vi "ComputeColorROI.vi"(1 "Array":dbl[](array[numeric])) -> (0 "Rectangle":T1 {"Rotation" min=-90.0 max=90.0 step=1.0 format="%.2f"; "Left" scale=0.0..1024.0; "Right" scale=0.0..1024.0})   [LabVIEW 2017]
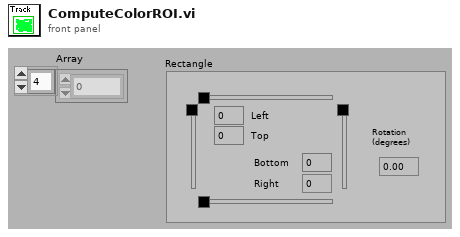
[diagram p1: front panel]
types:
  T1 = typedef "IMAQ Rectangle" = cluster{"Left":i32, "Top":i32, "Right":i32, "Bottom":i32, "Rotation":dbl}
  T2 = cluster{"Numeric":dbl, "Numeric":dbl, "Numeric":dbl, "Numeric":dbl}
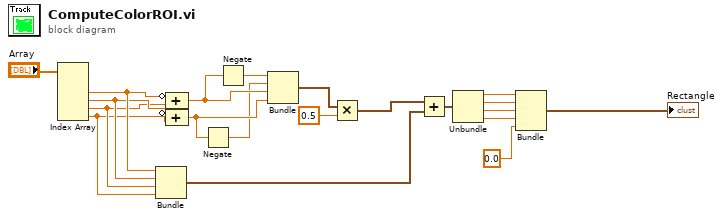
[diagram p0: block diagram]
diagram:
  n1 = Index Array(array="Array") -> (element #2=w10:dbl, element #3=w9:dbl, element #4=w8:dbl, element #5=w7:dbl)  [unwired: 5 in, 1 out]
  n2 = Bundle("Numeric"=w10, "Numeric"=w9, "Numeric"=w8, "Numeric"=w7) -> (w5:T2)  [unwired: 1 in]
  n3 = Compound Arithmetic op=ADD(invert w10, w8) -> (w15:dbl)
  n4 = Compound Arithmetic op=ADD(invert w9, w7) -> (w13:dbl)
  n5 = Negate(x=w13) -> (-x=w12:dbl)
  n6 = Negate(x=w15) -> (-x=w14:dbl)
  n7 = Bundle(w14, w12, w15, w13) -> (w11:cluster{dbl, dbl, dbl, dbl})  [unwired: 1 in]
  n8 = Multiply(x=w11, y=0.5) -> (x*y=w6:cluster{dbl, dbl, dbl, dbl})
  n9 = Add(x=w6, y=w5) -> (x+y=w20:cluster{dbl, dbl, dbl, dbl})
  n10 = Unbundle(w20) -> (w4:dbl, w3:dbl, w2:dbl, w1:dbl)
  n11 = Bundle(w4, w3, w2, w1, "y"=0.0) -> (→"Rectangle":cluster{dbl, dbl, dbl, dbl, "y":dbl})  [unwired: 1 in]
